vi "SBE37ExampleCopyWIP.vi"() -> ()   [LabVIEW 2023]
uses:
  <vilib>/Instr/_visa.llb/VISA Configure Serial Port (Instr).vi
panel:
  out "return count 3":u32
  in  "write buffer 2":string
  in  "millisecond timer value 3":u32
  out "return count 2":u32
  in  "byte count":u32
  in  "millisecond timer value 2":u32
  in  "filename":path
  out "VISA resource name out":refnum<visa-resource-name>
  out "return count":u32
  out "error out":errorcluster
  in  "write buffer":string
  in  "VISA resource name":refnum<visa-resource-name>
  in  "milliseconds to wait 3":u32
  in  "millisecond timer value":u32
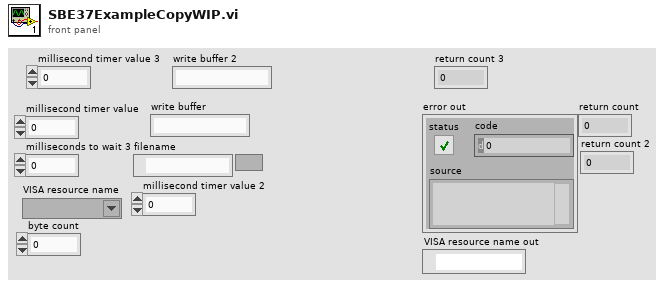
[diagram p1: front panel]
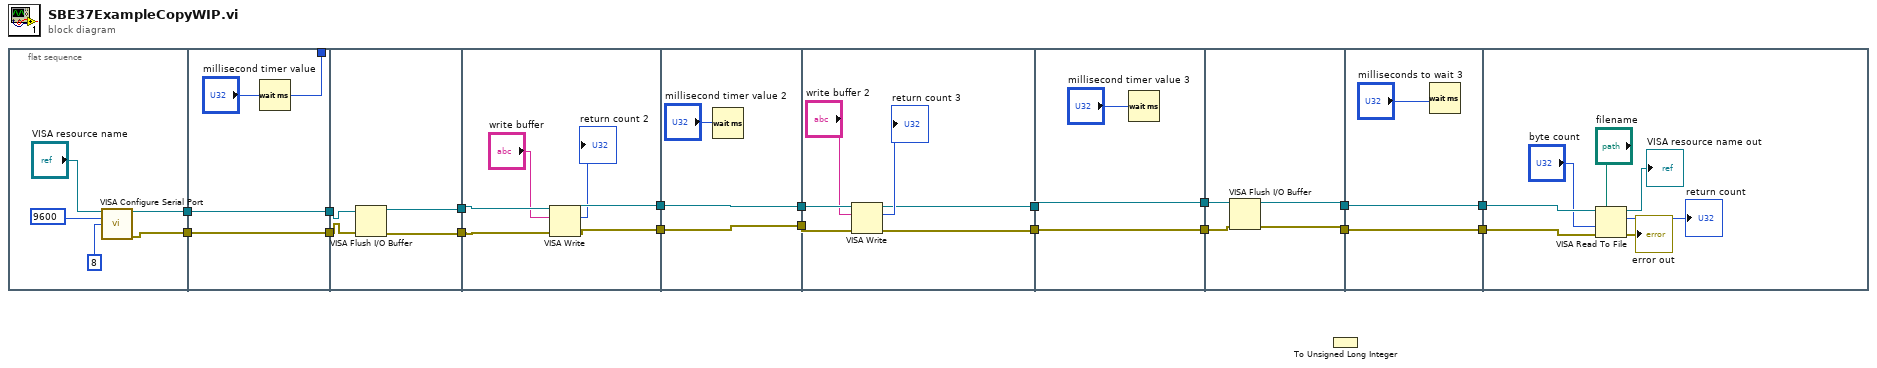
[diagram p0: block diagram]
diagram:
  n1 = flat-sequence {
    tunnel: [w21] -> w18
    tunnel: [w20] -> w17
    tunnel: w18 -> [w25]
    tunnel: w17 -> [w24]
    tunnel: [w26] -> _
    tunnel: [w25] -> w14
    tunnel: [w24] -> w13
    tunnel: [w29] -> w16
    tunnel: [w28] -> w15
    tunnel: w14 -> [w31]
    tunnel: w13 -> [w30]
    tunnel: w16 -> [w37]
    tunnel: w15 -> [w36]
    tunnel: [w35] -> w8
    tunnel: [w34] -> w7
    tunnel: w8 -> [w40]
    tunnel: [w40] -> w5
    tunnel: w7 -> [w39]
    tunnel: [w39] -> w4
    tunnel: w5 -> [w46]
    tunnel: w4 -> [w45]
    tunnel: [w44] -> w3
    tunnel: [w41] -> w2
    tunnel: w3 -> [w49]
    tunnel: [w49] -> w6
    tunnel: w2 -> [w47]
    tunnel: [w47] -> w1
    tunnel: [w53] -> w10
    tunnel: w6 -> [w52]
    tunnel: [w51] -> w9
    tunnel: w1 -> [w50]
    tunnel: w10 -> [w56]
    tunnel: [w56] -> w12
    tunnel: w9 -> [w55]
    tunnel: [w55] -> w11
    tunnel: w12 -> [w63]
    tunnel: w11 -> [w62]
    frame #0 {
      n2 = call-poly "VISA Configure Serial Port"("VISA resource name"="VISA resource name", "baud rate (9600)"=9600, "data bits (8)"=8) -> ("VISA resource name out"=w20:refnum<visa-resource-name>, "error out"=w21:errorcluster)  [unwired: 11 in]
    }
    frame #1 {
      n3 = Wait (ms)(milliseconds to wait="millisecond timer value") -> (millisecond timer value=w26:u32)
    }
    frame #2 {
      n4 = VISA Flush I/O Buffer(VISA resource name=w30, error in (no error)=w31) -> (VISA resource name out=w28:refnum<visa-resource-name>, error out=w29:errorcluster)  [unwired: 1 in]
    }
    frame #3 {
      n5 = VISA Write(VISA resource name=w36, write buffer="write buffer", error in (no error)=w37) -> (VISA resource name out=w35:refnum<visa-resource-name>, return count=→"return count 2":u32, error out=w34:errorcluster)
    }
    frame #4 {
      n6 = Wait (ms)(milliseconds to wait="millisecond timer value 2") -> ()  [unwired: 1 out]
    }
    frame #5 {
      n7 = VISA Write(VISA resource name=w46, write buffer="write buffer 2", error in (no error)=w45) -> (VISA resource name out=w41:refnum<visa-resource-name>, return count=→"return count 3":u32, error out=w44:errorcluster)
    }
    frame #6 {
      n8 = Wait (ms)(milliseconds to wait="millisecond timer value 3") -> ()  [unwired: 1 out]
    }
    frame #7 {
      n9 = VISA Flush I/O Buffer(VISA resource name=w50, error in (no error)=w52) -> (VISA resource name out=w53:refnum<visa-resource-name>, error out=w51:errorcluster)  [unwired: 1 in]
    }
    frame #8 {
      n10 = Wait (ms)(milliseconds to wait="milliseconds to wait 3") -> ()  [unwired: 1 out]
    }
    frame #9 {
      n11 = VISA Read To File(8:w62, 9:"byte count", 10:"filename", 11:w63) -> (0:→"error out":errorcluster, 2:→"return count":u32, 3:→"VISA resource name out":refnum<visa-resource-name>)
    }
  }
  n12 = To Unsigned Long Integer() -> ()  [unwired: 1 in, 1 out]
